vi "Agilent VNA Unflatten Driver Configuration.vi"(9 "VNA Configuration (\"\")":string) -> (1 "Configuration":T1={"BusType"=enum."GPIB", "GPIB Bus"=0, "GPIB Address"=0, "IP"=0, "COM"=0, "Baud Rate"=enum."300", "USB Device"=0, "Instrument S\\N"="", "SCIL Address"=16} {"USB Device" max=31 step=1}, 4 "Version":string)   [LabVIEW 2011]
uses:
  VNA Configuration.ctl
  VNA Configuration v1.ctl
  VNA Configuration v2.ctl
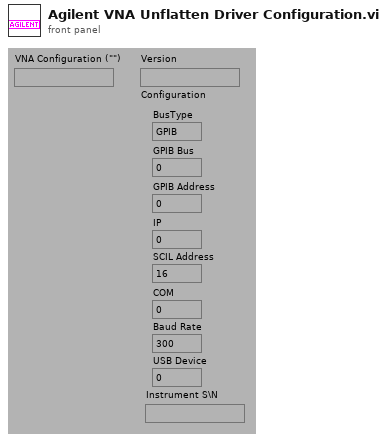
[diagram p1: front panel]
types:
  T1 = typedef "VNA Configuration.ctl" = cluster{"BusType":enum32{"GPIB", "LAN/IP", "Serial", "USB"}, "GPIB Bus":i32, "GPIB Address":i32, "IP":u32, "COM":i32, "Baud Rate":enum32{"300", "600", "1200", "2400", "4800", "9600"}, "USB Device":u32, "Instrument S\\N":string, "SCIL Address":i32}
  T2 = typedef "VNA Configuration v1.ctl" = cluster{"BusType":enum32{"GPIB", "LAN/IP", "Serial", "USB"}, "GPIB Bus":i32, "GPIB Address":i32, "IP":u32, "COM":i32, "Baud Rate":enum32{"300", "600", "1200", "2400", "4800", "9600"}}
  T3 = typedef "VNA Configuration v2.ctl" = cluster{"BusType":enum32{"GPIB", "LAN/IP", "Serial", "USB"}, "GPIB Bus":i32, "GPIB Address":i32, "IP":u32, "COM":i32, "Baud Rate":enum32{"300", "600", "1200", "2400", "4800", "9600"}, "USB Device":u32, "Instrument S\\N":string}
  T4 = enum32{"300", "600", "1200", "2400", "4800", "9600"}
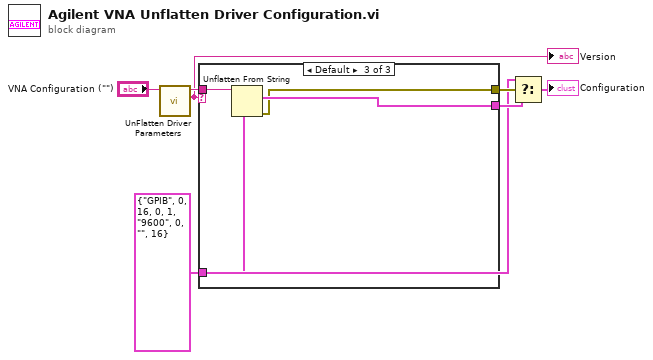
[diagram p0: block diagram]
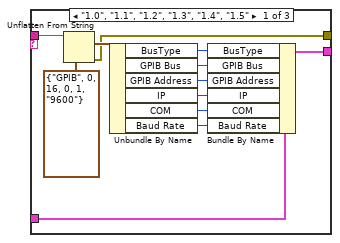
[diagram p2: hidden frame]
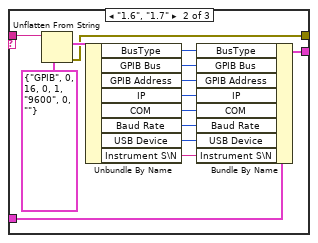
[diagram p3: hidden frame]
diagram:
  w2 = T1 {"BusType"=enum."GPIB", "GPIB Bus"=0, "GPIB Address"=16, "IP"=0, "COM"=1, "Baud Rate"=enum."9600", "USB Device"=0, "Instrument S\\N"="", "SCIL Address"=16} ("Configuration")
  n1 = call "UnFlatten Driver Parameters.vi"("Flattened Driver Parameters with Version (\"\")"="VNA Configuration (\"\")") -> ("Driver Version"=w1:string, "Flat Driver Parameters"=w3:string)  [unwired: 1 in, 4 out]
  "Version" <- w1
  n2 = case shown="Default" w1 {
    tunnel: [w16 w30 w37] -> w7
    tunnel: [w8 w20 w34] -> w5
    tunnel: w3 -> [w19 w33 w36]
    tunnel: w2 -> [w17 w31 w35]
    frame "1.0", "1.1", "1.2", "1.3", "1.4", "1.5" {
      n3 = Unflatten From String(type=T2 {"BusType"=enum."GPIB", "GPIB Bus"=0, "GPIB Address"=16, "IP"=0, "COM"=1, "Baud Rate"=enum."9600"} ("Configuration"), binary string=w19) -> (value=w15:T2, error out=w8:errorcluster)  [unwired: 1 in, 3 out]
      n4 = Unbundle By Name(w15) -> ("BusType"=w14:enum32{"GPIB", "LAN/IP", "Serial", "USB"}, "GPIB Bus"=w13:i32, "GPIB Address"=w12:i32, "IP"=w11:u32, "COM"=w10:i32, "Baud Rate"=w9:T4)
      n5 = Bundle By Name(cluster=w17, "BusType"=w14, "GPIB Bus"=w13, "GPIB Address"=w12, "IP"=w11, "COM"=w10, "Baud Rate"=w9) -> (w16:T1)
    }
    frame "1.6", "1.7" {
      n6 = Unflatten From String(type=T3 {"BusType"=enum."GPIB", "GPIB Bus"=0, "GPIB Address"=16, "IP"=0, "COM"=1, "Baud Rate"=enum."9600", "USB Device"=0, "Instrument S\\N"=""} ("Configuration"), binary string=w33) -> (value=w29:T3, error out=w20:errorcluster)  [unwired: 1 in, 3 out]
      n7 = Unbundle By Name(w29) -> ("BusType"=w28:enum32{"GPIB", "LAN/IP", "Serial", "USB"}, "GPIB Bus"=w27:i32, "GPIB Address"=w26:i32, "IP"=w25:u32, "COM"=w24:i32, "Baud Rate"=w23:T4, "USB Device"=w22:u32, "Instrument S\\N"=w21:string)
      n8 = Bundle By Name(cluster=w31, "BusType"=w28, "GPIB Bus"=w27, "GPIB Address"=w26, "IP"=w25, "COM"=w24, "Baud Rate"=w23, "USB Device"=w22, "Instrument S\\N"=w21) -> (w30:T1)
    }
    frame Default {
      n9 = Unflatten From String(type=w35, binary string=w36) -> (value=w37:T1, error out=w34:errorcluster)  [unwired: 1 in, 3 out]
    }
  }
  n10 = Select(t=w2, s=w5, f=w7) -> (s? t:f=→"Configuration":T1)
